vi "Periodic Tasks.vi"(8 "error in":errorcluster) -> (0 "error out":errorcluster)   [LabVIEW 2019]
doc: "This VI runs in parallel to other tasks. It can contain as many user-defined periodic loops as you need. These can carry out PID or other sorts of timed response."
uses:
  <vilib>/Rock Robotics/WPI/Ultrasonic/WPI_UltrasonicRangeUnits.ctl
  <vilib>/Rock Robotics/WPI/Ultrasonic/WPI_SonarSRF04DigitalRefNum Registry Get.vi
  <vilib>/Rock Robotics/WPI/Utilities/WPI_GetSetVariantRefNum.vi
  SubVi's/Global Sensors.vi
  <vilib>/Rock Robotics/WPI/Ultrasonic/WPI_SonarSRF04DigitalGetRange.vi
  <vilib>/Rock Robotics/Network Tables/NT Write Boolean.vi
  <vilib>/Rock Robotics/Network Tables/NT Write String.vi
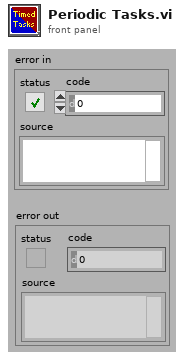
[diagram p1: front panel]
types:
  T1 = typedef "WPI_SwitchDevRef.ctl" = cluster{"DevStatus":errorcluster, "DIO Channel":T2, "CntIndex":T3, "Normally Closed":bool}
  T2 = typedef "FPGA_DIOChannel.ctl" = enum8{"DIO 0", "DIO 1", "DIO 2", "DIO 3", "DIO 4", "DIO 5", "DIO 6", "DIO 7", "DIO 8", "DIO 9", "DIO MXP 0", "DIO MXP 1", "DIO MXP 2", "DIO MXP 3", "DIO MXP 4", "DIO MXP 5", "DIO MXP 6", "DIO MXP 7", "DIO MXP 8", "DIO MXP 9", "DIO MXP 10", "DIO MXP 11", "DIO MXP 12", "DIO MXP 13", "DIO MXP 14", "DIO MXP 15", "SPI Port CS1", "SPI Port CS2", "SPI Port CS3", "SPI Port MISO", "SPI Port MOSI", "Invalid"}
  T3 = typedef "FPGA_CounterCtrSystemIndex.ctl" = enum8{"Ctr 0", "Ctr 1", "Ctr 2", "Ctr 3", "Ctr 4", "Ctr 5", "Ctr 6", "Ctr 7", "Invalid"}
  T4 = typedef "WPI_CompressorDevRef.ctl" = cluster{"DevStatus":errorcluster, "Pneumatics Control Module":u8}
  T5 = typedef "Color Sensor V3 DevRef.ctl" = cluster{"I2CDevRef":T6}
  T6 = typedef "WPI_I2CDevRef.ctl" = cluster{"DevStatus":errorcluster, "Device Address":u8, "Handle":i32, "I2C Bus":T7}
  T7 = typedef "i2c_bus.ctl" = enum16{"I2C On-Board", "I2C MXP", "Invalid"}
  T8 = typedef "WPI_UltrasonicDeviceRef.ctl" = cluster{"DevStatus":errorcluster, "Ping Channel":T2, "Echo Channel":T2, "CntIndex":T3}
  T9 = typedef "WPI_UltrasonicRangeUnits.ctl" = enum16{"inches", "mm"}
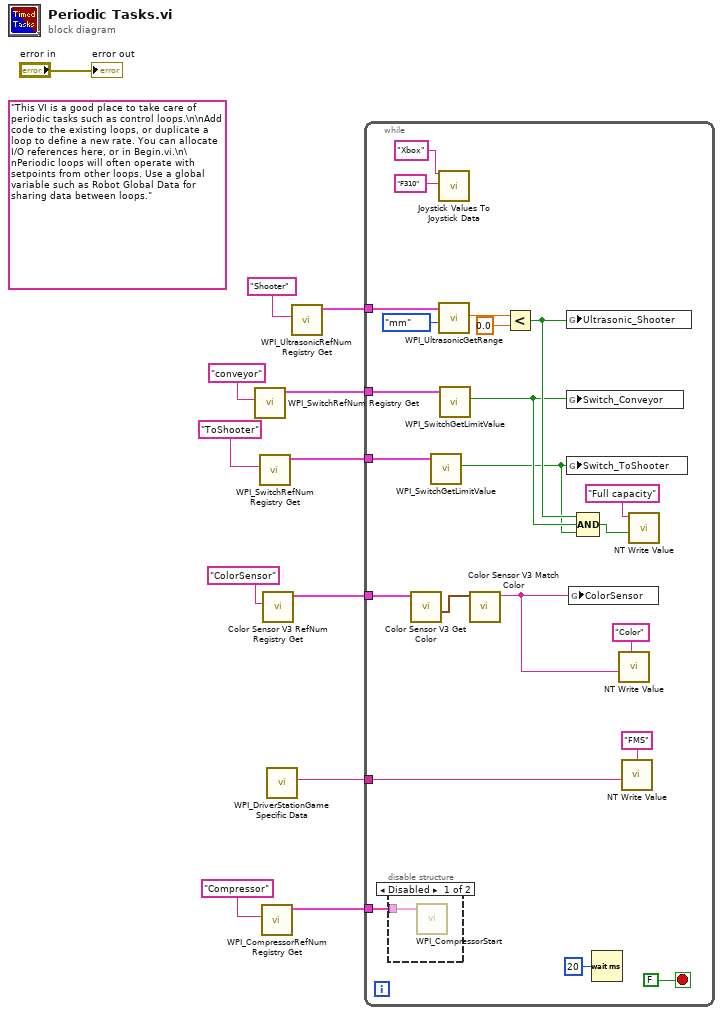
[diagram p0: block diagram]
diagram:
  (unwired) "This VI is a good place to take care of periodic tasks such as control loops.\n\nAdd code to the existing loops, or duplicate a loop to define a new rate. You can allocate I/O references here, or in Begin.vi.\n\nPeriodic loops will often operate with setpoints from other loops. Use a global variable such as Robot Global Data for sharing data between loops."
  n1 = call <vilib>:"WPI_SwitchRefNum Registry Get.vi"("refnum name"="conveyor") -> ("SwitchDevRef"=w9:T1)  [unwired: 9 in, 1 out]
  n2 = call <vilib>:"WPI_SwitchRefNum Registry Get.vi"("refnum name"="ToShooter") -> ("SwitchDevRef"=w3:T1)  [unwired: 9 in, 1 out]
  n3 = call <vilib>:"WPI_CompressorRefNum Registry Get.vi"("refnum name"="Compressor") -> ("CompressorDevRef"=w5:T4)  [unwired: 9 in, 1 out]
  n4 = call <vilib>:"Color Sensor V3 RefNum Registry Get.vi"("refnum name"="ColorSensor") -> ("ColorSensorDevRef"=w7:T5)  [unwired: 9 in, 1 out]
  n5 = call <vilib>:"WPI_DriverStationGame Specific Data.vi"() -> ("Game Specific Data"=w1:string)  [unwired: 11 in]
  n6 = call-poly <vilib>:"WPI_UltrasonicRefNum Registry Get.vi"("refnum name"="Shooter") -> ("SonarSRF04DevRef"=w11:T8)  [unwired: 9 in, 1 out]
  n7 = while {
    tunnel: w11 -> [w31]
    tunnel: w9 -> [w27]
    tunnel: w7 -> [w26]
    tunnel: w5 -> [w24]
    tunnel: w3 -> [w23]
    tunnel: w1 -> [w13]
    stop <- FALSE stop-if-true
    n8 = disable-structure shown="Disabled" {
      disable-tunnel: w24 -> [w35 _]
      frame Disabled {
        n9 = call <vilib>:"WPI_CompressorStart.vi"("CompressorDevRef"=w35) -> ()  [unwired: 9 in, 2 out]
      }
      frame Enabled {
      }
    }
    n10 = call <vilib>:"Color Sensor V3 Get Color.vi"("ColorSensorDevRef"=w26) -> ("Normalized Color"=w25:cluster{"R":dbl, "G":dbl, "B":dbl})  [unwired: 7 in, 3 out]
    n11 = call <vilib>:"WPI_SwitchGetLimitValue.vi"("SwitchDevRef"=w23) -> ("Switch Pressed"=w19:bool)  [unwired: 8 in, 2 out]
    n12 = call "Joystick Values To Joystick Data.vi"("Xbox Name"="Xbox", "F310 Name"="F310") -> ()  [unwired: 18 in]
    n13 = call-poly <vilib>:"WPI_UltrasonicGetRange.vi"("Range Units"=WPI_UltrasonicRangeUnits."mm", "SonarSRF04DevRef"=w31) -> ("Distance"=w29:dbl)  [unwired: 7 in, 2 out]
    n14 = call <vilib>:"WPI_SwitchGetLimitValue.vi"("SwitchDevRef"=w27) -> ("Switch Pressed"=w20:bool)  [unwired: 8 in, 2 out]
    n15 = call <vilib>:"Color Sensor V3 Match Color.vi"("Measured Color"=w25) -> ("Matched Color Name"=w16:string)  [unwired: 8 in, 2 out]
    n16 = Less?(x=w29, y=0.0) -> (x < y?=w21:bool)
    n17 = global write "Global Sensors.vi" "Ultrasonic_Shooter"(w21) -> ()
    n18 = global write "Global Sensors.vi" "Switch_Conveyor"(w20) -> ()
    n19 = global write "Global Sensors.vi" "Switch_ToShooter"(w19) -> ()
    n20 = global write "Global Sensors.vi" "ColorSensor"(w16) -> ()
    n21 = Compound Arithmetic op=AND(w21, w20, w19) -> (w18:bool)
    n22 = Wait (ms)(milliseconds to wait=u32 20) -> ()  [unwired: 1 out]
    n23 = call-poly <vilib>:"NT Write Value.vi"("String"=w16, "Name"="Color") -> ()  [unwired: 9 in, 1 out]
    n24 = call-poly <vilib>:"NT Write Value.vi"("String"=w13, "Name"="FMS") -> ()  [unwired: 9 in, 1 out]
    n25 = call-poly <vilib>:"NT Write Value.vi"("Boolean"=w18, "Name"="Full capacity") -> ()  [unwired: 9 in, 1 out]
  }
  "error out" <- "error in"
